vi "Node Format.vi"(8 "error in":errorcluster, 10 "Node (0-64)":i8 min=0 max=64 step=1) -> (0 "error out":errorcluster, 2 "Formatted Node":string)   [LabVIEW 2013, in "Keithley 2600 Series.lvlib"]
doc: "This VI wil format a string for use with the <b>Node In</b> parameter of other VIs in the instrument driver."
uses:
  Keithley 2600 Series.lvlib
panel:
  # "(c) 2008 Keithley Instruments, Inc.  ALL RIGHTS RESERVED."
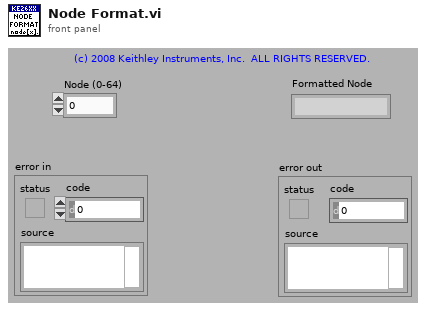
[diagram p1: front panel]
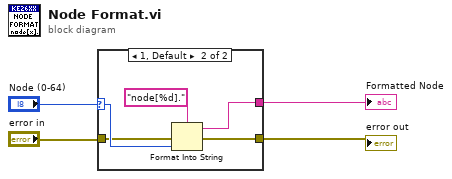
[diagram p0: block diagram]
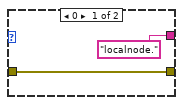
[diagram p2: hidden frame]
diagram:
  n1 = case shown="1, Default" "Node (0-64)" {
    selector: "Node (0-64)" -> [_ w10]
    tunnel: ["localnode." w9] -> w3
    tunnel: "error in" -> [w6 w8]
    tunnel: [w6 w7] -> w1
    frame 0 {
    }
    frame 1, Default {
      n2 = Format Into String(format string="node[%d].", error in=w8, w10) -> (resulting string=w9:string, error out=w7:errorcluster)  [unwired: 1 in]
    }
  }
  "Formatted Node" <- w3
  "error out" <- w1
